vi "Perform_AFP.vi"(7 "AFP Efficiency":dbl, 8 "AFP Target":i32, 9 "rho-":dbl[](array[numeric]), 10 "rho0":dbl[](array[numeric]), 11 "rho+":dbl[](array[numeric])) -> (1 "rho- out":dbl[](array[numeric]), 2 "rho0 out":dbl[](array[numeric]), 3 "rho+ out":dbl[](array[numeric]))   [LabVIEW 2018]
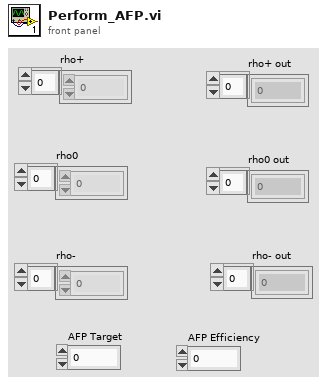
[diagram p1: front panel]
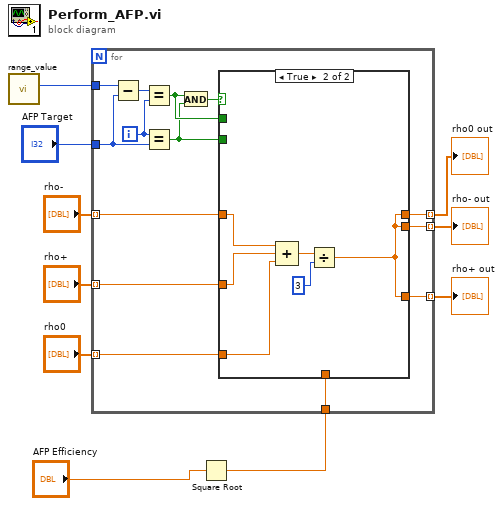
[diagram p0: block diagram]
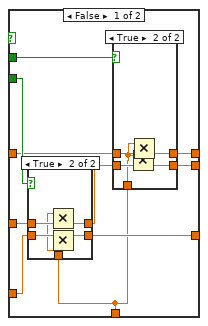
[diagram p2: hidden frame]
diagram:
  n1 = call "range_value.vi"() -> ("NumBins"=w3:i32)  [unwired: 10 in, 1 out]
  n2 = Square Root(x="AFP Efficiency") -> (sqrt(x)=w1:dbl)
  n3 = for {
    tunnel: "rho+" -> [w17] mode=indexing
    tunnel: "rho0" -> [w16] mode=indexing
    tunnel: "rho-" -> [w15] mode=indexing
    tunnel: w3 -> [w24]
    tunnel: "AFP Target" -> [w21]
    tunnel: [w14] -> w6 mode=indexing
    tunnel: [w13] -> w5 mode=indexing
    tunnel: [w12] -> w4 mode=indexing
    tunnel: w1 -> [w11]
    i -> [w22]
    n4 = Subtract(x=w24, y=w21) -> (x-y=w23:i32)
    n5 = Equal?(x=w23, y=w22) -> (x = y?=w20:bool)
    n6 = Equal?(x=w22, y=w21) -> (x = y?=w18:bool)
    n7 = And(x=w20, y=w18) -> (x .and. y?=w19:bool)
    n8 = case shown="True" w19 {
      tunnel: w20 -> [w34 _]
      tunnel: w18 -> [w33 _]
      tunnel: w17 -> [w32 w53]
      tunnel: w16 -> [w31 w52]
      tunnel: [w29 w49] -> w14
      tunnel: w15 -> [w28 w54]
      tunnel: [w27 w49] -> w12
      tunnel: [w26 w49] -> w13
      tunnel: w11 -> [w25 _]
      frame False {
        n9 = case shown="True" w33 {
          tunnel: w32 -> [w36 w41]
          tunnel: w31 -> [w35 w40]
          tunnel: [w36 w39] -> w29
          tunnel: [w35 w38] -> w30
          tunnel: w25 -> [_ w37]
          frame False {
          }
          frame True {
            n10 = Multiply(x=w37, y=w41) -> (x*y=w38:dbl)
            n11 = Multiply(x=w40, y=w37) -> (x*y=w39:dbl)
          }
        }
        n12 = case shown="True" w34 {
          tunnel: w30 -> [w43 w48]
          tunnel: [w43 w46] -> w26
          tunnel: w28 -> [w42 w47]
          tunnel: [w42 w45] -> w27
          tunnel: w25 -> [_ w44]
          frame False {
          }
          frame True {
            n13 = Multiply(x=w44, y=w48) -> (x*y=w45:dbl)
            n14 = Multiply(x=w44, y=w47) -> (x*y=w46:dbl)
          }
        }
      }
      frame True {
        n15 = Compound Arithmetic op=ADD(w54, w53, w52) -> (w51:dbl)
        n16 = Divide(x=w51, y=3) -> (x/y=w49:dbl)
      }
    }
  }
  "rho+ out" <- w6
  "rho0 out" <- w5
  "rho- out" <- w4
